vi "Drive Motor Read Values.vi"(6 "Configuration":T2={"Accelerometer Bias"={"X (m/s)"=0.0, "Y (m/s)"=0.0, "Z (m/s)"=0.0}, "Gyroscope Bias"={"X (m/s)"=0.0, "Y (m/s)"=0.0, "Z (m/s)"=0.0}, "Steering Motor Gear Ratio"=611.0, "Steering Pully Gear Ratio"=1.0, "Steering Encoder CPR"=500.0, "Steering Motor Max RPM"=4000.0, "Wheelbase (m)"=1.12, "Fork Angle (rad)"=1.3, "Balancing Controller"={"Kp (/s)"=0.0, "Kd (1)"=0.0}, "Max Allowed Steering Angle (rad)"=0.7, "Task Periods"={"Emergency Stop (us)"=0, "IMU (us)"=0, "Steering Motor Encoder (us)"=0, "State Estimator (us)"=0, "Balancing Controller (us)"=0, "GNSS (us)"=0, "Logging (us)"=0, "Drive Motor (us)"=0}, "Drive Motor Gear Ratio"=0.7, "Drive Motor UART Delay (ms)"=10}, 8 "Controller Data In":refnum<data-value>, 10 "Drive Motor Handle In":T1, 11 "Error In":errorcluster) -> (0 "Controller Data Out":refnum<data-value>, 1 "Drive Motor Data":T3, 2 "Drive Motor Handle Out":T1, 3 "Error Out":errorcluster)   [LabVIEW 2021]
uses:
  Drive Motor Handle.ctl
  Drive Motor Data.ctl
  Configuration/Configuration.ctl
  Logging/Controller Data.ctl
  Steering Motor/Steering Motor Data.ctl
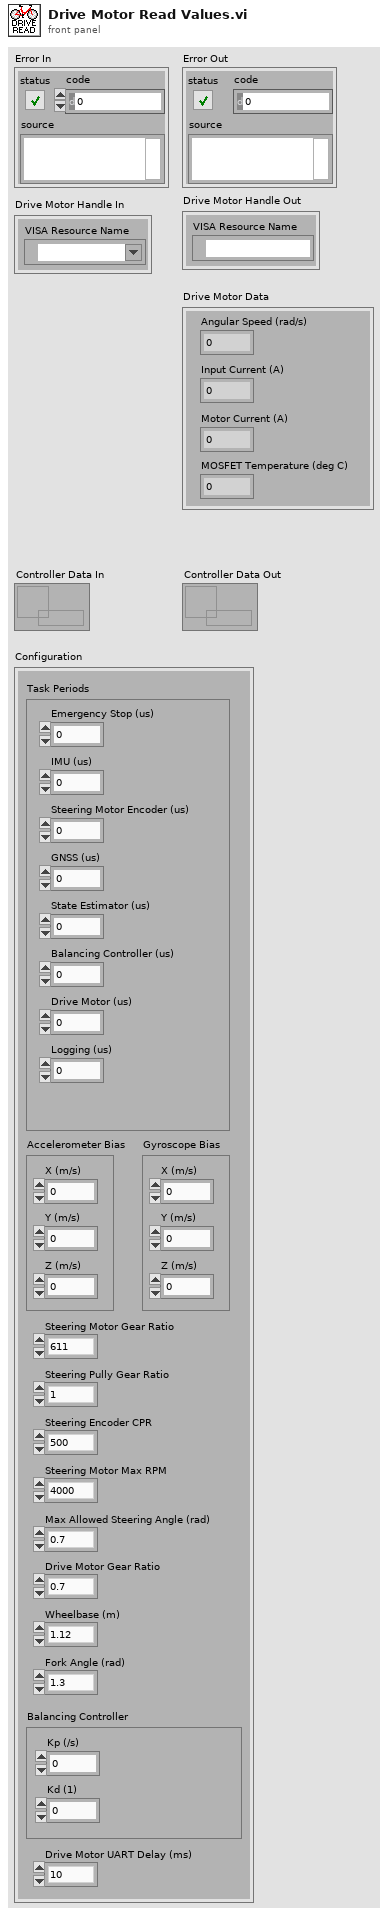
[diagram p1: front panel]
types:
  T1 = typedef "Drive Motor Handle.ctl" = cluster{"VISA Resource Name":refnum<visa-resource-name>}
  T2 = typedef "Configuration.ctl" = cluster{"Accelerometer Bias":cluster{"X (m/s)":dbl, "Y (m/s)":dbl, "Z (m/s)":dbl}, "Gyroscope Bias":cluster{"X (m/s)":dbl, "Y (m/s)":dbl, "Z (m/s)":dbl}, "Steering Motor Gear Ratio":dbl, "Steering Pully Gear Ratio":dbl, "Steering Encoder CPR":dbl, "Steering Motor Max RPM":dbl, "Wheelbase (m)":dbl, "Fork Angle (rad)":dbl, "Balancing Controller":cluster{"Kp (/s)":dbl, "Kd (1)":dbl}, "Max Allowed Steering Angle (rad)":dbl, "Task Periods":cluster{"Emergency Stop (us)":i64, "IMU (us)":i64, "Steering Motor Encoder (us)":i64, "State Estimator (us)":i64, "Balancing Controller (us)":i64, "GNSS (us)":i64, "Logging (us)":i64, "Drive Motor (us)":i64}, "Drive Motor Gear Ratio":dbl, "Drive Motor UART Delay (ms)":i64}
  T3 = typedef "Drive Motor Data.ctl" = cluster{"Angular Speed (rad/s)":dbl, "Input Current (A)":dbl, "Motor Current (A)":dbl, "MOSFET Temperature (deg C)":dbl}
  T4 = typedef "Controller Data.ctl" = cluster{"Drive Motor Data":T3, "Steering Motor Data":T5}
  T5 = typedef "Steering Motor Data.ctl" = cluster{"PWM":dbl, "Steering Angle Rate (rad/s)":dbl}
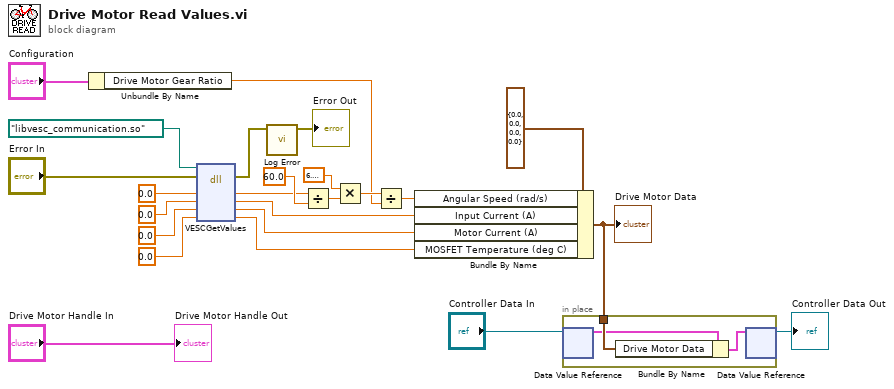
[diagram p0: block diagram]
diagram:
  n1 = Unbundle By Name("Configuration") -> ("Drive Motor Gear Ratio"=w8:dbl)
  n2 = dll-call lib="?" fn="VESCGetValues"(path in=path "libvesc_communication.so", error in="Error In", "RPM"=0.0, "currentIn"=0.0, "currentMotor"=0.0 ("RPM"), "tempMOS"=0.0 ("currentIn")) -> (error out=w14:errorcluster, "RPM"=w12:dbl, "currentIn"=w11:dbl, "currentMotor"=w16:dbl, "tempMOS"=w1:dbl)  [unwired: 2 in, 1 out]
  n3 = call "Log Error.vi"("Error In"=w14) -> ("Error Out"=→"Error Out":errorcluster)  [unwired: 10 in]
  n4 = Divide(x=w12, y=60.0 ("x")) -> (x/y=w18:dbl)
  n5 = Multiply(x=6.283185307179586, y=w18) -> (x*y=w9:dbl)
  n6 = Divide(x=w9, y=w8) -> (x/y=w7:dbl)
  n7 = Bundle By Name(cluster=T3 {"Angular Speed (rad/s)"=0.0, "Input Current (A)"=0.0, "Motor Current (A)"=0.0, "MOSFET Temperature (deg C)"=0.0} ("Drive Motor Data"), "Angular Speed (rad/s)"=w7, "Input Current (A)"=w11, "Motor Current (A)"=w16, "MOSFET Temperature (deg C)"=w1) -> (w3:T3)
  "Drive Motor Data" <- w3
  n8 = in-place {
    in-place-border: w3 -> [w26]
    n9 = in-place-dvr #1("Controller Data In") -> (w25:T4)  [unwired: 1 out]
    n10 = Bundle By Name(cluster=w25, "Drive Motor Data"=w26) -> (w27:T4)
    n11 = in-place-dvr #1(w27) -> (→"Controller Data Out":refnum<data-value>)  [unwired: 1 out]
  }
  "Drive Motor Handle Out" <- "Drive Motor Handle In"
